vi "DHE_AdjustTimeout.vi"(9 "old exptime":dbl, 10 "new exptime":dbl) -> ()   [LabVIEW 2016]
uses:
  SCL_Action.ctl
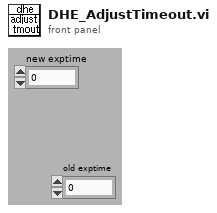
[diagram p1: front panel]
types:
  T1 = typedef "SCL_Action.ctl" = enum16{"Add", "Callback", "Shutdown", "modif timeout", "delete", "delete async"}
  T2 = typedef "SCL_Pending Action.ctl" = cluster{"Cmd Ref":i32, "Dev Ref":string, "TimeOut":i32, "TimeInit":i32, "CallbackVI":string, "Link Ref":string}
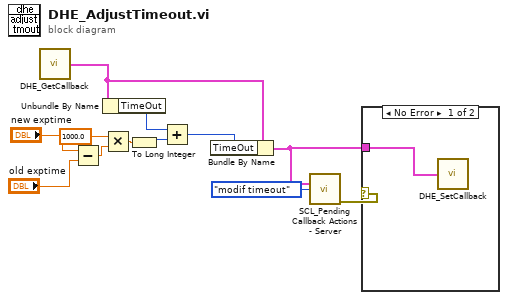
[diagram p0: block diagram]
diagram:
  n1 = call "DHE_GetCallback.vi"() -> ("DHE_CallBack"=w1:T2)  [unwired: 9 in]
  n2 = Subtract(x="new exptime", y="old exptime") -> (x-y=w6:dbl)
  n3 = Unbundle By Name(w1) -> ("TimeOut"=w9:i32)
  n4 = Multiply(x=1000.0, y=w6) -> (x*y=w7:dbl)
  n5 = To Long Integer(number=w7) -> (32bit integer=w2:i32)
  n6 = Add(x=w9, y=w2) -> (x+y=w8:i32)
  n7 = Bundle By Name(cluster=w1, "TimeOut"=w8) -> (w3:T2)
  n8 = call "SCL_Pending Callback Actions - Server.vi"("Pending Callback"=w3, "Action"=SCL_Action."modif timeout") -> ("error out"=w4:errorcluster)  [unwired: 13 in]
  n9 = case shown="No Error" w4 {
    tunnel: w3 -> [w13 _]
    frame No Error {
      n10 = call "DHE_SetCallback.vi"("DHE_CallBack"=w13) -> ()  [unwired: 9 in]
    }
    frame Error {
    }
  }
